vi "Fit-1.vi"() -> ()   [LabVIEW 2012]
uses:
  <vilib>/Utility/file.llb/Read From Spreadsheet File (DBL).vi
panel:
  in  "Path":path
  out "XY Graph":cluster{"all rows":dbl[], "all rows":dbl[]}(graph)
  out "all rows":dbl[][](array[numeric]) format="%0.3f"
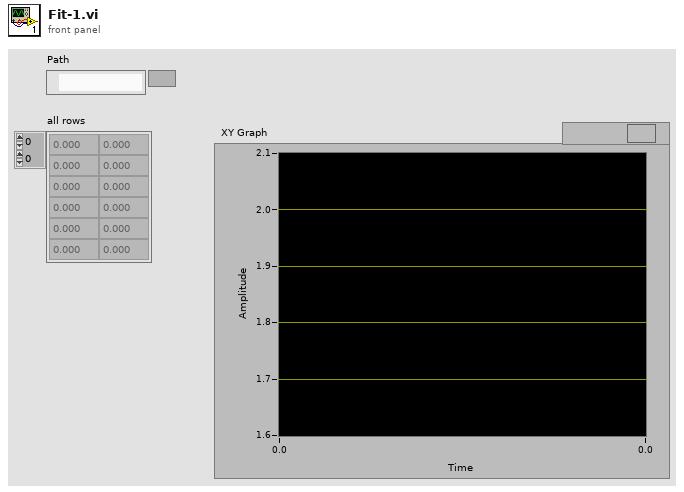
[diagram p1: front panel]
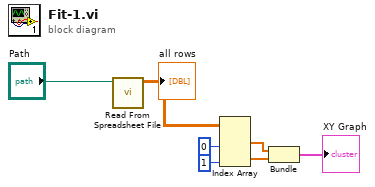
[diagram p0: block diagram]
diagram:
  n1 = call-poly <vilib>:"Read From Spreadsheet File.vi"("file path (dialog if empty)"="Path") -> ("all rows"=w7:dbl[][])  [unwired: 6 in, 4 out]
  "all rows" <- w7
  n2 = Index Array(array=w7, index (col) #1=0 ("disabled index (col)"), index (col) #2=1 ("index (col)")) -> (element #1=w6:dbl[], element #2=w5:dbl[])  [unwired: 2 in]
  n3 = Bundle("all rows"=w6, "all rows"=w5) -> (→"XY Graph":cluster{"all rows":dbl[], "all rows":dbl[]})  [unwired: 1 in]
